vi "MovemotorMengXYMain2.vi"(5 "dir":dbl[](array[numeric]), 6 "Joystick axis":i32, 7 "Motor settings (X,Y)":cluster{"Vmax (mm/s)":sgl, "Acc (mm/s/s)":sgl}={"Vmax (mm/s)"=0.1, "Acc (mm/s/s)"=0.05}, 8 "error in (no error)":errorcluster, 9 "XorYMAX":sgl, 10 "XorYMIN":sgl, 11 "Automation Refnum in":refnum<k7>) -> (0 "error out":errorcluster, 2 "Automation Refnum out":refnum<k7>, 3 "XorYPosition":sgl, 4 "dir 2":dbl[](array[numeric]))   [LabVIEW 2014]
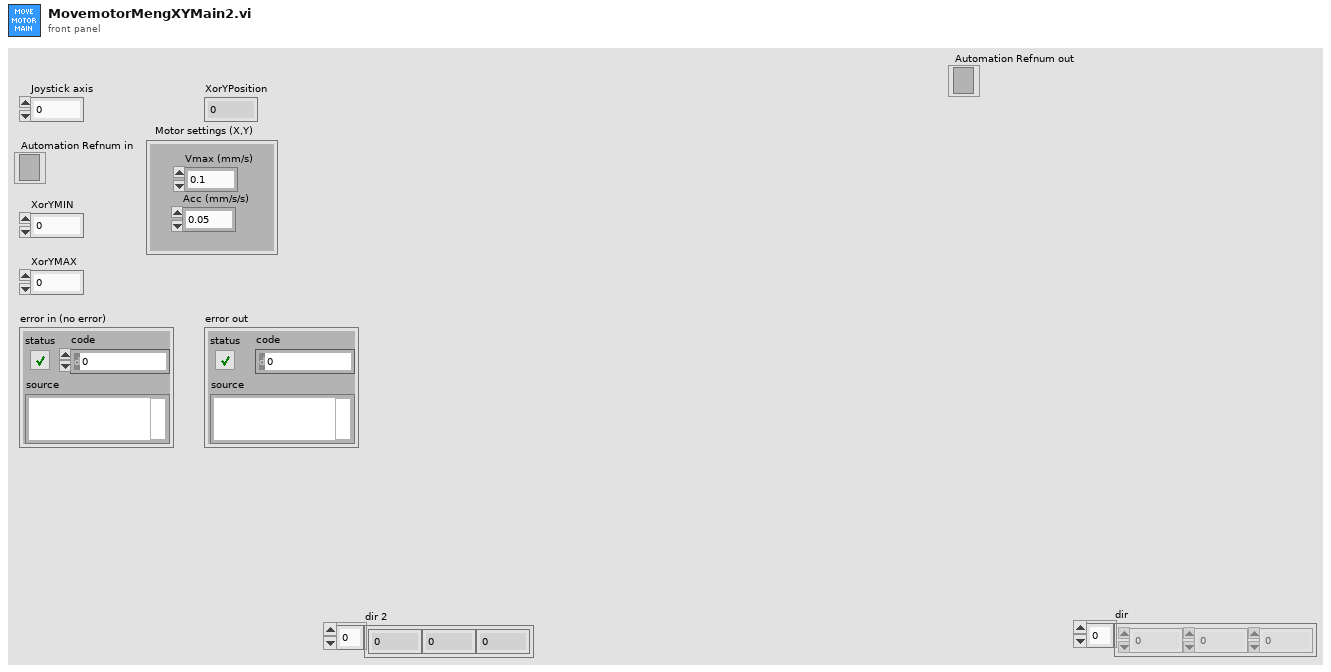
[diagram p1: front panel]
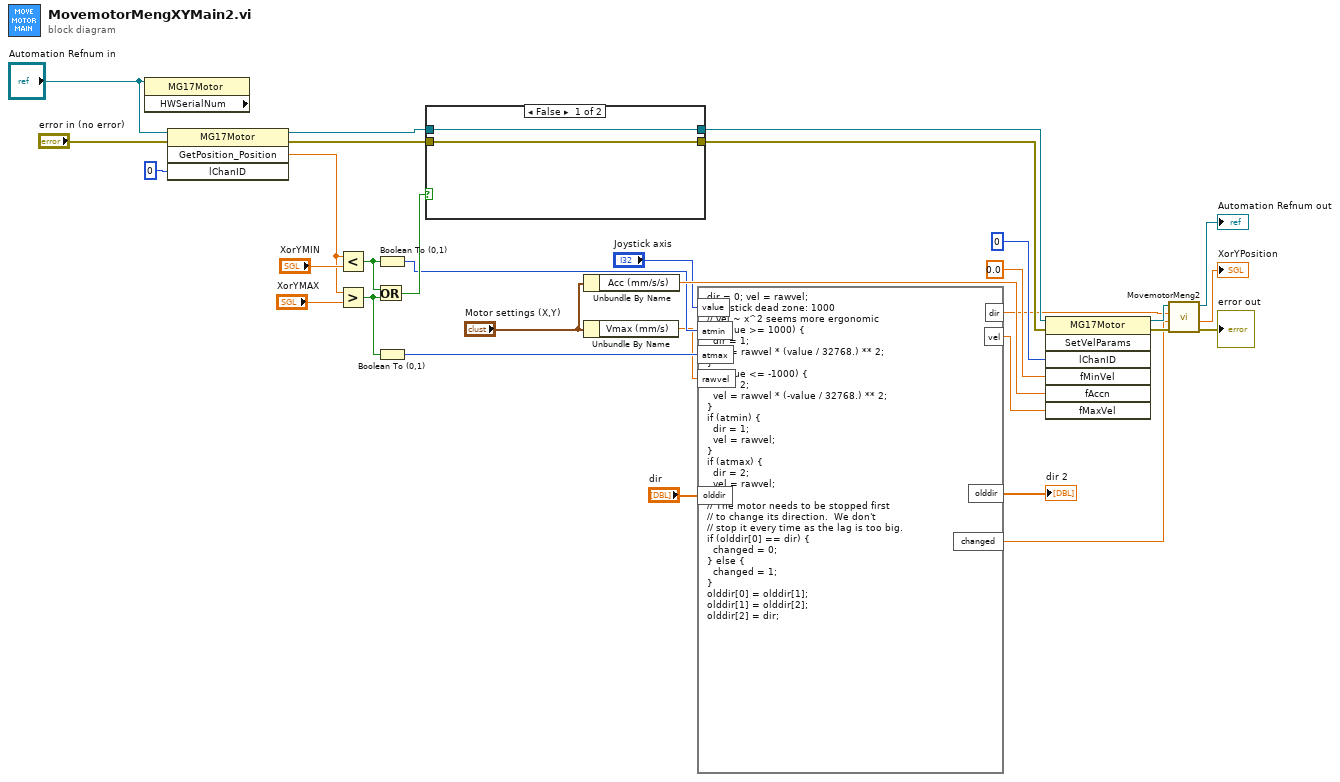
[diagram p0: block diagram]
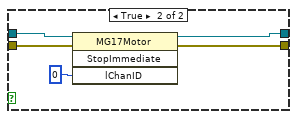
[diagram p2: hidden frame]
diagram:
  n1 = property class="MG17Motor" props=["HWSerialNum"](reference="Automation Refnum in") -> ()  [unwired: 1 in, 3 out]
  n2 = invoke class="MG17Motor" method="GetPosition_Position"(reference="Automation Refnum in", error in="error in (no error)", "lChanID"=0) -> (reference out=w30:refnum<k7>, error out=w29:errorcluster, "GetPosition_Position"=w25:sgl)  [unwired: 1 in, 1 out]
  n3 = Less?(x=w25, y="XorYMIN") -> (x < y?=w10:bool)
  n4 = Greater?(x=w25, y="XorYMAX") -> (0:w21:bool)
  n5 = Or(x=w10, y=w21) -> (x .or. y?=w28:bool)
  n6 = Boolean To (0,1)(Boolean=w10) -> (0, 1=w9:i16)
  n7 = Boolean To (0,1)(Boolean=w21) -> (0, 1=w8:i16)
  n8 = case shown="False" w28 {
    tunnel: w30 -> [w33 w38]
    tunnel: w29 -> [w32 w37]
    tunnel: [w32 w36] -> w13
    tunnel: [w33 w35] -> w14
    frame False {
    }
    frame True {
      n9 = invoke class="MG17Motor" method="StopImmediate"(reference=w38, error in=w37, "lChanID"=0) -> (reference out=w35:refnum<k7>, error out=w36:errorcluster)  [unwired: 1 in, 2 out]
    }
  }
  n10 = Unbundle By Name("Motor settings (X,Y)") -> ("Acc (mm/s/s)"=w19:sgl)
  n11 = Unbundle By Name("Motor settings (X,Y)") -> ("Vmax (mm/s)"=w7:sgl)
  n12 = formula code="dir = 0; vel = rawvel;\n// Joystick dead zone: 1000\n// vel ~ x^2 seems more ergonomic\nif (value >= 1000) {\n  dir = 1;\n  vel = rawvel * (value / 32768.) ** 2;\n}\nif (value <= -1000) {\n  dir = 2;\n  vel = rawvel * (-value / 32768.) ** 2;\n}\nif (atmin) {\n  dir = 1;\n  vel = rawvel;\n}\nif (atmax) {\n  dir = 2;\n  vel = rawvel;\n}\n// The motor needs to be stopped first\n// to change its direction.  We don't\n// stop it every time as the lag is too big.\nif (olddir[0] == dir) {\n  changed = 0;\n} else {\n  changed = 1;\n}\nolddir[0] = olddir[1];\nolddir[1] = olddir[2];\nolddir[2] = dir;"("value"="Joystick axis", "atmin"=w9, "atmax"=w8, "rawvel"=w7, "olddir"="dir") -> ("dir"=w4:dbl, "vel"=w6:dbl, "olddir"=→"dir 2":dbl[], "changed"=w1:dbl)
  n13 = invoke class="MG17Motor" method="SetVelParams"(reference=w14, error in=w13, "lChanID"=0, "fMinVel"=0.0 ("lChanID"), "fAccn"=w19, "fMaxVel"=w6) -> (reference out=w15:refnum<k7>, error out=w12:errorcluster)  [unwired: 1 in, 5 out]
  n14 = call "MovemotorMeng2.vi"("error in (no error)"=w12, "change"=w1, "direction"=w4, "Automation Refnum in"=w15) -> ("error out"=→"error out":errorcluster, "Position"=→"XorYPosition":sgl, "Automation Refnum out"=→"Automation Refnum out":refnum<k7>)  [unwired: 5 in]
